vi "autolock.vi"   [LabVIEW 2012]
uses:
  <vilib>/Rock Robotics/WPI/Relay/WPI_RelayValue.ctl
  Robot Global Data.vi
  <vilib>/Rock Robotics/WPI/RobotDrive/WPI_RobotDriveGetSetRefNum.vi
types:
  T1 = typedef "WPI_RelayDevRef.ctl" = cluster{"DevStatus":errorcluster, "Relay Channel":T2, "Digital Module":T3, "Relay Direction":T4}
  T2 = typedef "FPGA_DIORelayChannel.ctl" = enum8{"Relay 1", "Relay 2", "Relay 3", "Relay 4", "Relay 5", "Relay 6", "Relay 7", "Relay 8", "Invalid"}
  T3 = typedef "FPGA_TypedefDigitalModule.ctl" = enum16{"Digital Module 1", "Digital Module 2"}
  T4 = typedef "WPI_RelayDirection.ctl" = enum16{"Both directions", "Forward only", "Reverse only"}
  T5 = typedef "WPI_RelayValue.ctl" = enum16{"Off", "On", "Forward", "Reverse"}
  T6 = cluster{"Position":cluster{"X":i32, "Y":i32}, "Distance (ft)":i32, "Center":bool, "Top":bool, "Mid":bool}
  T7 = cluster{"Center Position":cluster{"X":dbl, "Y":dbl}, "Distance (ft)":dbl, "Center":bool, "Top":bool, "Mid":bool}[]
  T8 = typedef "WPI_RobotDriveDevRef.ctl" = cluster{"DevStatus":errorcluster, "Motors[]":T9[], "Square Inputs":bool, "Max Output":dbl, "Isochronous":bool}
  T9 = typedef "WPI_MotorControlDeviceRef.ctl" = cluster{"DeviceStatus":errorcluster, "Type":enum16{"PWM", "CAN"}, "PWM":cluster{"Digital Module":T3, "PWM Channel":T10, "DeadBand":T11}, "CAN":cluster{"Device Number":u8, "Control Mode":T12, "Semaphore":T13, "Max Vout":dbl}, "Invert":bool, "TransformRef":T14, "InvTransformRef":T14}
  T10 = typedef "FPGA_DIOPWMChannel.ctl" = enum8{"PWM 1", "PWM 2", "PWM 3", "PWM 4", "PWM 5", "PWM 6", "PWM 7", "PWM 8", "PWM 9", "PWM 10", "Invalid"}
  T11 = typedef "WPI_PWMDeadband.ctl" = cluster{"Name":string, "maxPositivePwm":i32, "minPositivePwm":i32, "centerPwm":i32, "maxNegativePwm":i32, "minNegativePwm":i32, "angularRange":u16}
  T12 = typedef "WPI_CANJaguar_ControlMode.ctl" = enum8{"Percent VBus", "Current", "Speed", "Position", "Voltage"}
  T13 = typedef "Semaphore RefNum" = refnum<k1>
  T14 = typedef "WPI_PWMTransform_ConPane.ctl" = refnum<vi>
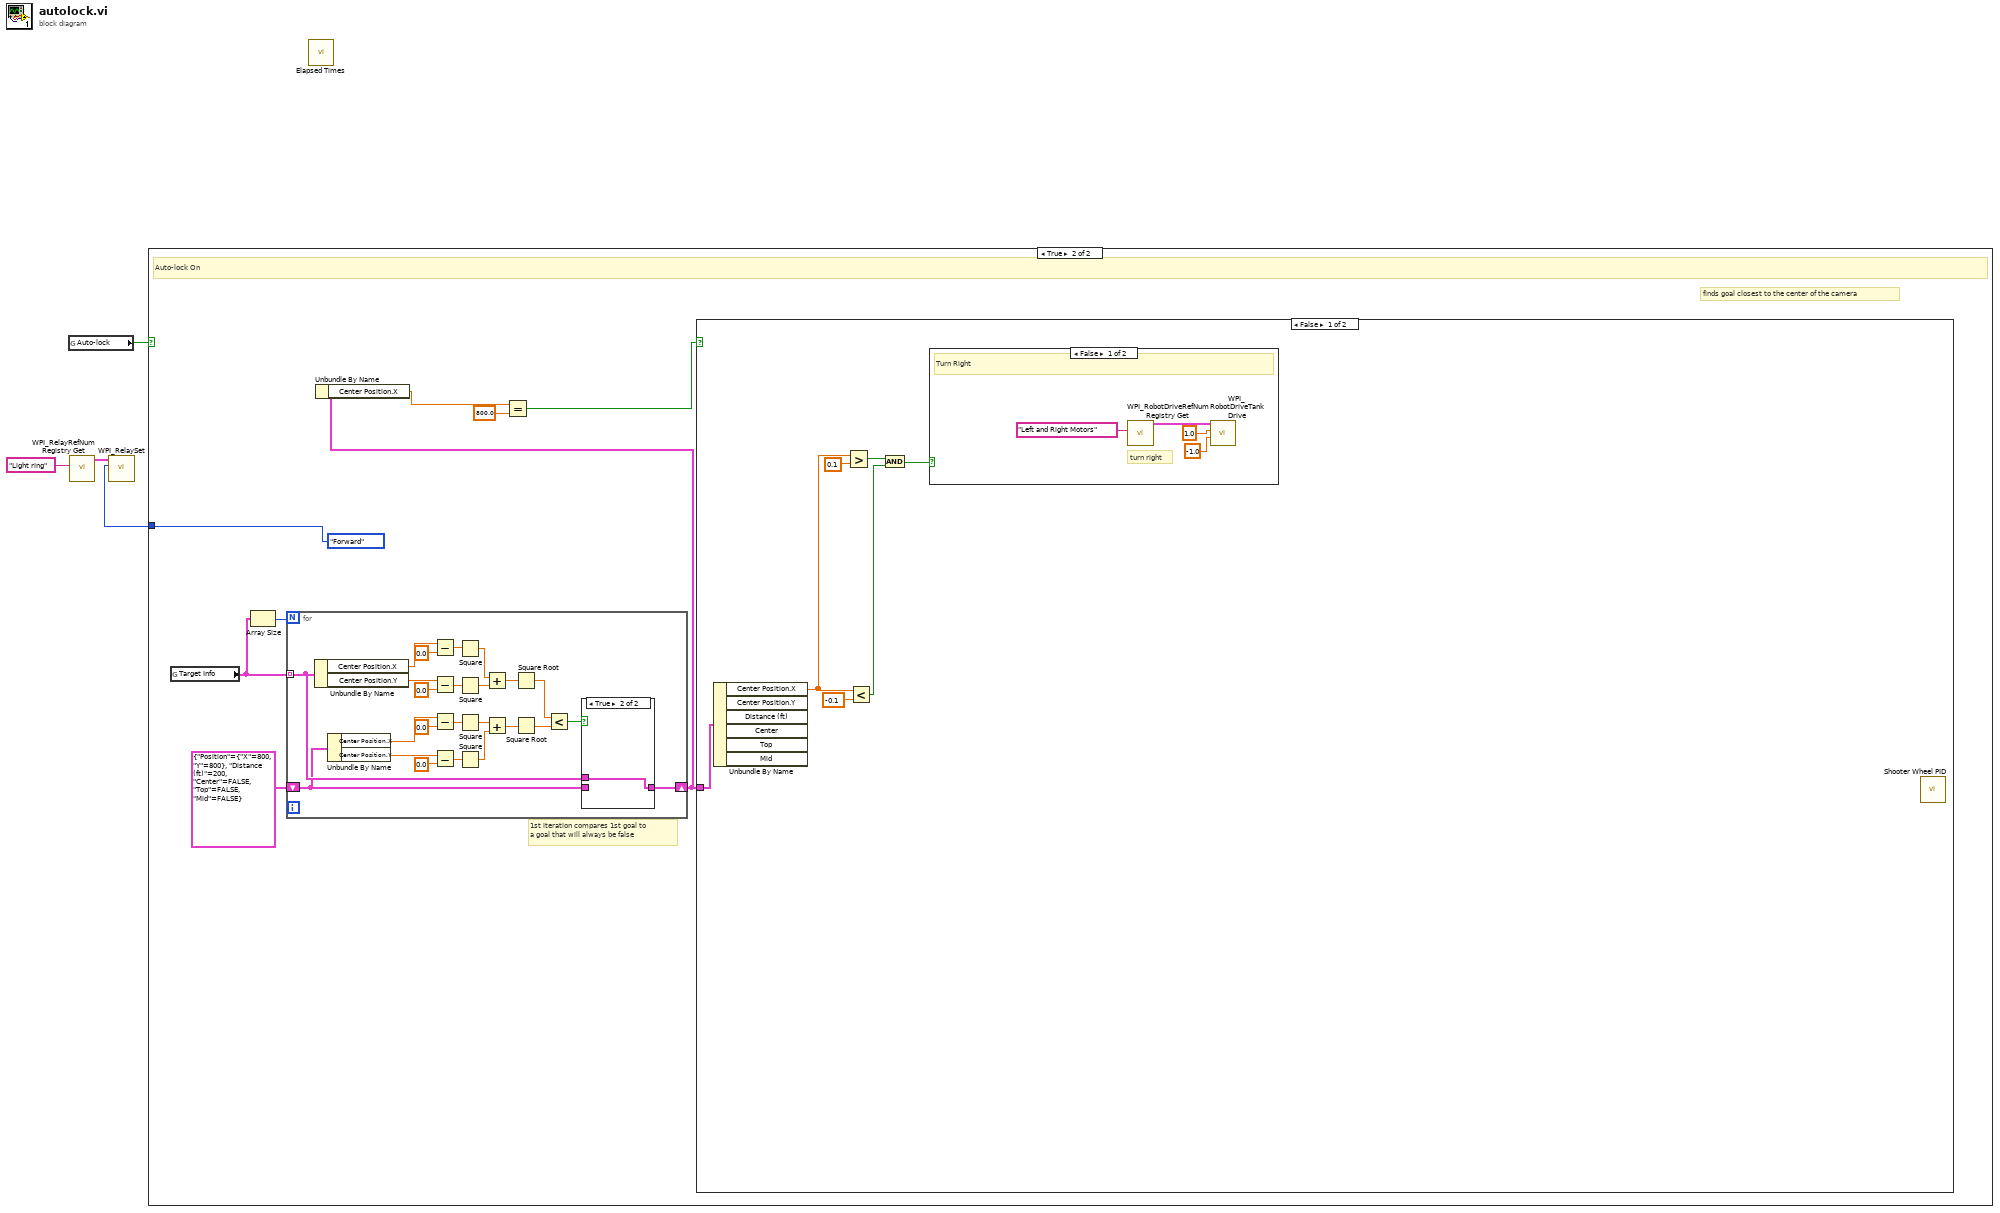
[diagram p0: block diagram]
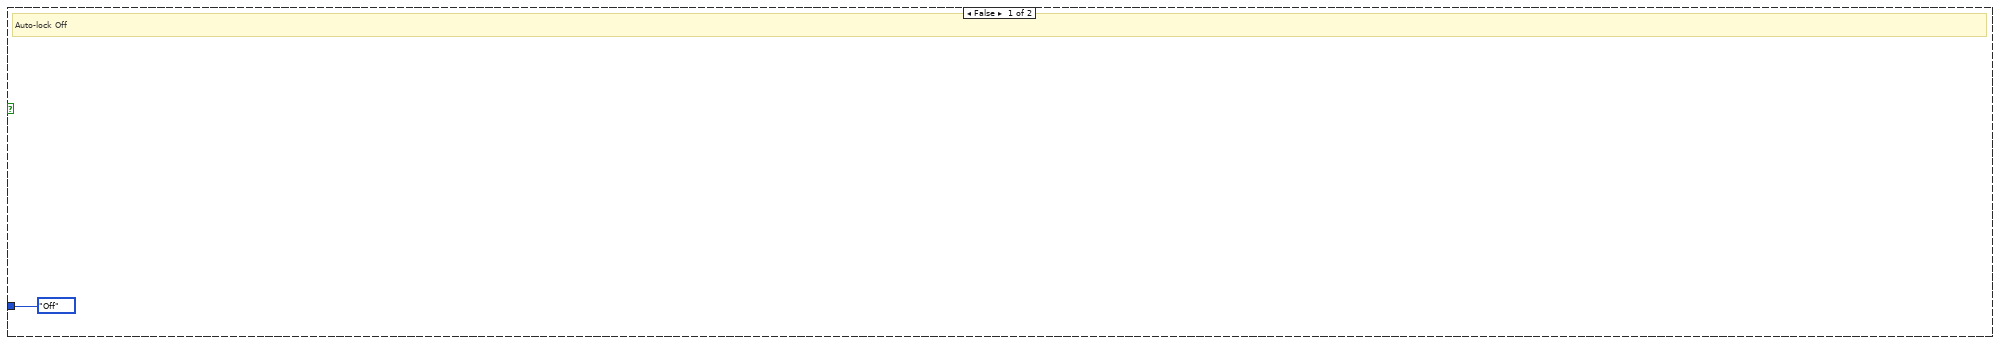
[diagram p2: hidden frame]
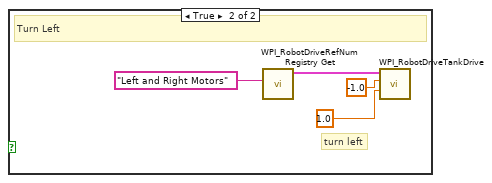
[diagram p3: hidden frame]
diagram:
  n1 = global read "Robot Global Data.vi" "Auto-lock"() -> (w4:bool)
  n2 = call <vilib>:"WPI_RelayRefNum Registry Get.vi"("refnum name"="Light ring") -> ("RelayDevRef"=w2:T1)  [unwired: 9 in, 1 out]
  n3 = case shown="True" w4 {
    tunnel: [WPI_RelayValue."Off" ("RelayValue") WPI_RelayValue."Forward" ("RelayValue")] -> w1
    frame False {
      # "Auto-lock Off"
    }
    frame True {
      # "1st iteration compares 1st goal to \na goal that will always be false"
      # "finds goal closest to the center of the camera"
      # "Auto-lock On"
      n4 = global read "Robot Global Data.vi" "Target Info"() -> (w12:T7)
      n5 = Array Size(array=w12) -> (size(s)=w13:i32)
      n6 = for {
        N: w13 -> [_]
        tunnel: w12 -> [w44] mode=indexing
        shift-right: [w43] -> w9
        shift-left: T6 {"Position"={"X"=800, "Y"=800}, "Distance (ft)"=200, "Center"=FALSE, "Top"=FALSE, "Mid"=FALSE} -> [w42]
        n7 = Unbundle By Name(w44) -> ("Center Position.X"=w29:dbl, "Center Position.Y"=w33:dbl)
        n8 = Unbundle By Name(w42) -> ("Center Position.X"=w40:dbl, "Center Position.Y"=w37:dbl)
        n9 = Subtract(x=w29, y=0.0) -> (x-y=w30:dbl)
        n10 = Subtract(x=w33, y=0.0) -> (x-y=w32:dbl)
        n11 = Subtract(x=w40, y=0.0) -> (x-y=w38:dbl)
        n12 = Subtract(x=w37, y=0.0) -> (x-y=w35:dbl)
        n13 = Square(x=w30) -> (x^2=w50:dbl)
        n14 = Square(x=w32) -> (x^2=w49:dbl)
        n15 = Square(x=w38) -> (x^2=w48:dbl)
        n16 = Square(x=w35) -> (x^2=w47:dbl)
        n17 = Add(x=w50, y=w49) -> (x+y=w52:dbl)
        n18 = Add(x=w48, y=w47) -> (x+y=w51:dbl)
        n19 = Square Root(x=w52) -> (sqrt(x)=w46:dbl)
        n20 = Square Root(x=w51) -> (sqrt(x)=w45:dbl)
        n21 = Less?(x=w46, y=w45) -> (x < y?=w41:bool)
        n22 = case shown="True" w41 {
          tunnel: w44 -> [_ w54]
          tunnel: [w53 w54] -> w43
          tunnel: w42 -> [w53 _]
          frame False {
          }
          frame True {
          }
        }
      }
      n23 = Unbundle By Name(w9) -> ("Center Position.X"=w8:dbl)
      n24 = Equal?(x=w8, y=800.0) -> (x = y?=w11:bool)
      n25 = case shown="False" w11 {
        tunnel: w9 -> [w15 _]
        frame False {
          n26 = Unbundle By Name(w15) -> ("Center Position.X"=w14:dbl)  [unwired: 5 out]
          n27 = Greater?(x=w14, y=0.1) -> (0:w17:bool)
          n28 = Less?(x=w14, y=-0.1) -> (x < y?=w18:bool)
          n29 = And(x=w17, y=w18) -> (x .and. y?=w16:bool)
          n30 = case shown="False" w16 {
            frame False {
              # "turn right"
              # "Turn Right"
              n31 = call <vilib>:"WPI_RobotDriveRefNum Registry Get.vi"("refnum name"="Left and Right Motors") -> ("RobotDriveDevRef"=w21:T8)  [unwired: 1 in, 9 out]
              n32 = call <vilib>:"WPI_RobotDriveTankDrive.vi"("Right axis value"=-1.0, "Left axis value"=1.0, "RobotDriveDevRef"=w21) -> ()  [unwired: 6 in, 3 out]
            }
            frame True {
              # "turn left"
              # "Turn Left"
              n33 = call <vilib>:"WPI_RobotDriveRefNum Registry Get.vi"("refnum name"="Left and Right Motors") -> ("RobotDriveDevRef"=w25:T8)  [unwired: 1 in, 9 out]
              n34 = call <vilib>:"WPI_RobotDriveTankDrive.vi"("Right axis value"=1.0, "Left axis value"=-1.0, "RobotDriveDevRef"=w25) -> ()  [unwired: 6 in, 3 out]
            }
          }
          n35 = call "Shooter Wheel PID.vi"() -> ()  [unwired: 11 in]
        }
        frame True {
        }
      }
    }
  }
  n36 = call <vilib>:"WPI_RelaySet.vi"("RelayValue"=w1, "RelayDevRef"=w2) -> ()  [unwired: 8 in, 2 out]
  n37 = call "Elapsed Times.vi"() -> ()  [unwired: 3 in, 1 out]
